vi "Calculatte DCAP_Percentage.vi"(6 "Data2 In":string, 8 "Error In":errorcluster, 9 "Target Cap (fF)":dbl, 11 "Data1 In":string) -> (0 "Error Out":errorcluster, 3 "Delta  C(fF)":string, 4 "% Delta C":string)   [LabVIEW 2017]
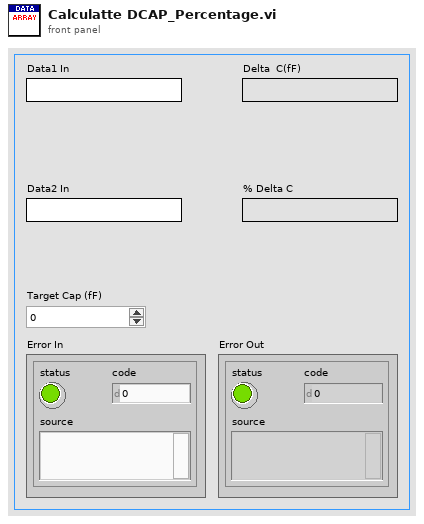
[diagram p1: front panel]
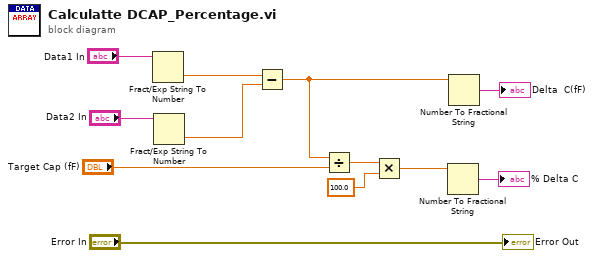
[diagram p0: block diagram]
diagram:
  n1 = Fract/Exp String To Number(string="Data1 In") -> (number=w11:dbl)  [unwired: 3 in, 1 out]
  n2 = Fract/Exp String To Number(string="Data2 In") -> (number=w9:dbl)  [unwired: 3 in, 1 out]
  n3 = Subtract(x=w11, y=w9) -> (x-y=w8:dbl)
  n4 = Divide(x=w8, y="Target Cap (fF)") -> (x/y=w2:dbl)
  n5 = Multiply(x=w2, y=100.0) -> (x*y=w3:dbl)
  n6 = Number To Fractional String(number=w3) -> (F-format string=→"% Delta C":string)  [unwired: 3 in]
  n7 = Number To Fractional String(number=w8) -> (F-format string=→"Delta  C(fF)":string)  [unwired: 3 in]
  "Error Out" <- "Error In"
